vi "WILT Update State.vi"(10 "Station Number":i32, 11 "Station Test State In in":T1) -> (3 "Station Test State In out":T1)   [LabVIEW 2016]
uses:
  Type Definitions/WILT Station Test State Cluster.ctl
  Type Definitions/WILT Dryer Test State.ctl
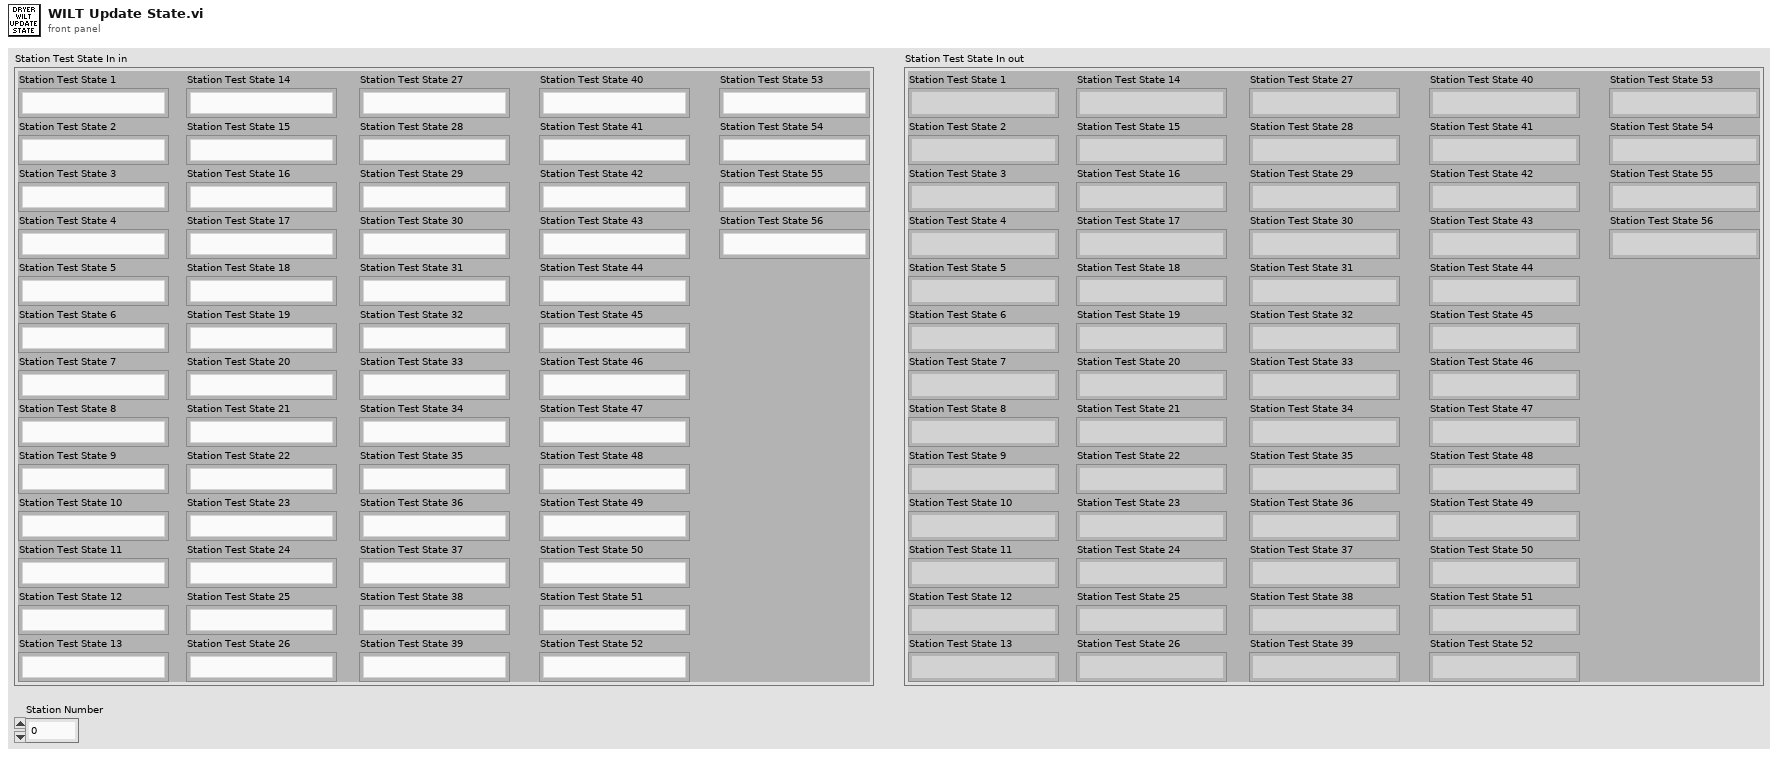
[diagram p1: front panel]
types:
  T1 = typedef "WILT Station Test State Cluster.ctl" = cluster{"Station Test State 1":T2, "Station Test State 2":T2, "Station Test State 3":T2, "Station Test State 4":T2, "Station Test State 5":T2, "Station Test State 6":T2, "Station Test State 7":T2, "Station Test State 8":T2, "Station Test State 9":T2, "Station Test State 10":T2, "Station Test State 11":T2, "Station Test State 12":T2, "Station Test State 13":T2, "Station Test State 14":T2, "Station Test State 15":T2, "Station Test State 16":T2, "Station Test State 17":T2, "Station Test State 18":T2, "Station Test State 19":T2, "Station Test State 20":T2, "Station Test State 21":T2, "Station Test State 22":T2, "Station Test State 23":T2, "Station Test State 24":T2, "Station Test State 25":T2, "Station Test State 26":T2, "Station Test State 27":T2, "Station Test State 28":T2, "Station Test State 29":T2, "Station Test State 30":T2, "Station Test State 31":T2, "Station Test State 32":T2, "Station Test State 33":T2, "Station Test State 34":T2, "Station Test State 35":T2, "Station Test State 36":T2, "Station Test State 37":T2, "Station Test State 38":T2, "Station Test State 39":T2, "Station Test State 40":T2, "Station Test State 41":T2, "Station Test State 42":T2, "Station Test State 43":T2, "Station Test State 44":T2, "Station Test State 45":T2, "Station Test State 46":T2, "Station Test State 47":T2, "Station Test State 48":T2, "Station Test State 49":T2, "Station Test State 50":T2, "Station Test State 51":T2, "Station Test State 52":T2, "Station Test State 53":T2, "Station Test State 54":T2, "Station Test State 55":T2, "Station Test State 56":T2}
  T2 = typedef "WILT Dryer Test State.ctl" = enum16{"No Serial Number", "Waiting for Dryer To Start", "Drying Clothes", "Water Injection 1 (On)", "Water Injection 1 Timer", "Water Injection 1 (Off)", "Pause Dryer", "Sending Start Stop CMD", "Pause Dryer 2", "Sending Start Stop CMD 2", "Drying Clothes 2", "Water Injection 2 (On)", "Water Injection 2 Timer", "Water Injection 2 (Off)", "Drying Clothes 3", "Cooling Down", "Sending Start Stop CMD 3", "Increment Cycle"}
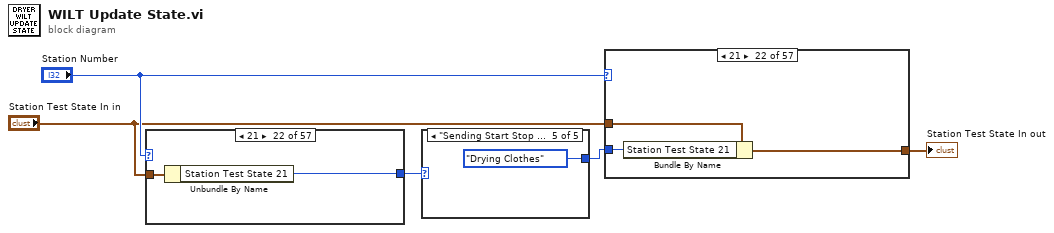
[diagram p0: block diagram]
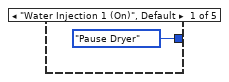
[diagram p2: hidden frame]
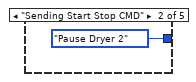
[diagram p3: hidden frame]
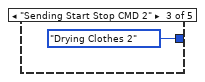
[diagram p4: hidden frame]
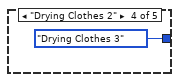
[diagram p5: hidden frame]
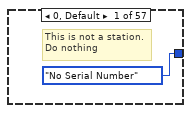
[diagram p6: hidden frame]
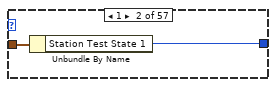
[diagram p7: hidden frame]
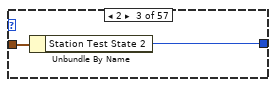
[diagram p8: hidden frame]
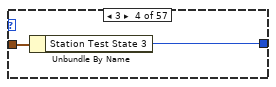
[diagram p9: hidden frame]
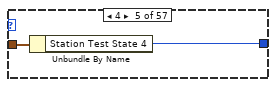
[diagram p10: hidden frame]
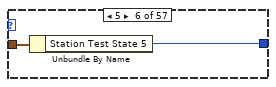
[diagram p11: hidden frame]
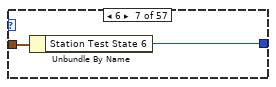
[diagram p12: hidden frame]
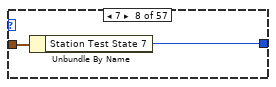
[diagram p13: hidden frame]
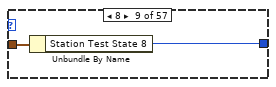
[diagram p14: hidden frame]
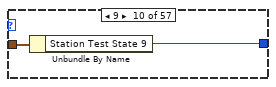
[diagram p15: hidden frame]
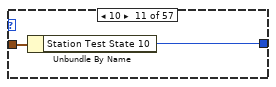
[diagram p16: hidden frame]
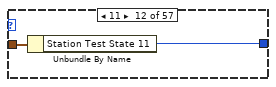
[diagram p17: hidden frame]
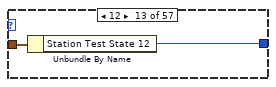
[diagram p18: hidden frame]
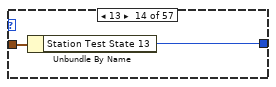
[diagram p19: hidden frame]
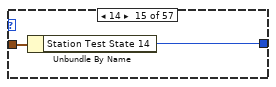
[diagram p20: hidden frame]
diagram:
  n1 = case shown="21" "Station Number" {
    tunnel: "Station Test State In in" -> [_ w8 w10 w12 w14 w16 w18 w20 w22 w24 w26 w28 w30 w32 w34 w36 w38 w40 w42 w44 w46 w48 w50 w52 w54 w56 w58 w60 w62 w64 w66 w68 w70 w72 w74 w76 w78 w80 w82 w84 w86 w88 w90 w92 w94 w96 w98 w100 w102 w104 w106 w108 w110 w112 w114 w116 w118]
    tunnel: [WILT_Dryer_Test_State."No Serial Number" ("Station Test State 56") w7 w9 w11 w13 w15 w17 w19 w21 w23 w25 w27 w29 w31 w33 w35 w37 w39 w41 w43 w45 w47 w49 w51 w53 w55 w57 w59 w61 w63 w65 w67 w69 w71 w73 w75 w77 w79 w81 w83 w85 w87 w89 w91 w93 w95 w97 w99 w101 w103 w105 w107 w109 w111 w113 w115 w117] -> w2
    frame 0, Default {
      # "This is not a station.\nDo nothing"
    }
    frame 1 {
      n2 = Unbundle By Name(w8) -> ("Station Test State 1"=w7:T2)
    }
    frame 2 {
      n3 = Unbundle By Name(w10) -> ("Station Test State 2"=w9:T2)
    }
    frame 3 {
      n4 = Unbundle By Name(w12) -> ("Station Test State 3"=w11:T2)
    }
    frame 4 {
      n5 = Unbundle By Name(w14) -> ("Station Test State 4"=w13:T2)
    }
    frame 5 {
      n6 = Unbundle By Name(w16) -> ("Station Test State 5"=w15:T2)
    }
    frame 6 {
      n7 = Unbundle By Name(w18) -> ("Station Test State 6"=w17:T2)
    }
    frame 7 {
      n8 = Unbundle By Name(w20) -> ("Station Test State 7"=w19:T2)
    }
    frame 8 {
      n9 = Unbundle By Name(w22) -> ("Station Test State 8"=w21:T2)
    }
    frame 9 {
      n10 = Unbundle By Name(w24) -> ("Station Test State 9"=w23:T2)
    }
    frame 10 {
      n11 = Unbundle By Name(w26) -> ("Station Test State 10"=w25:T2)
    }
    frame 11 {
      n12 = Unbundle By Name(w28) -> ("Station Test State 11"=w27:T2)
    }
    frame 12 {
      n13 = Unbundle By Name(w30) -> ("Station Test State 12"=w29:T2)
    }
    frame 13 {
      n14 = Unbundle By Name(w32) -> ("Station Test State 13"=w31:T2)
    }
    frame 14 {
      n15 = Unbundle By Name(w34) -> ("Station Test State 14"=w33:T2)
    }
    frame 15 {
      n16 = Unbundle By Name(w36) -> ("Station Test State 15"=w35:T2)
    }
    frame 16 {
      n17 = Unbundle By Name(w38) -> ("Station Test State 16"=w37:T2)
    }
    frame 17 {
      n18 = Unbundle By Name(w40) -> ("Station Test State 17"=w39:T2)
    }
    frame 18 {
      n19 = Unbundle By Name(w42) -> ("Station Test State 18"=w41:T2)
    }
    frame 19 {
      n20 = Unbundle By Name(w44) -> ("Station Test State 19"=w43:T2)
    }
    frame 20 {
      n21 = Unbundle By Name(w46) -> ("Station Test State 20"=w45:T2)
    }
    frame 21 {
      n22 = Unbundle By Name(w48) -> ("Station Test State 21"=w47:T2)
    }
    frame 22 {
      n23 = Unbundle By Name(w50) -> ("Station Test State 22"=w49:T2)
    }
    frame 23 {
      n24 = Unbundle By Name(w52) -> ("Station Test State 23"=w51:T2)
    }
    frame 24 {
      n25 = Unbundle By Name(w54) -> ("Station Test State 24"=w53:T2)
    }
    frame 25 {
      n26 = Unbundle By Name(w56) -> ("Station Test State 25"=w55:T2)
    }
    frame 26 {
      n27 = Unbundle By Name(w58) -> ("Station Test State 26"=w57:T2)
    }
    frame 27 {
      n28 = Unbundle By Name(w60) -> ("Station Test State 27"=w59:T2)
    }
    frame 28 {
      n29 = Unbundle By Name(w62) -> ("Station Test State 28"=w61:T2)
    }
    frame 29 {
      n30 = Unbundle By Name(w64) -> ("Station Test State 29"=w63:T2)
    }
    frame 30 {
      n31 = Unbundle By Name(w66) -> ("Station Test State 30"=w65:T2)
    }
    frame 31 {
      n32 = Unbundle By Name(w68) -> ("Station Test State 31"=w67:T2)
    }
    frame 32 {
      n33 = Unbundle By Name(w70) -> ("Station Test State 32"=w69:T2)
    }
    frame 33 {
      n34 = Unbundle By Name(w72) -> ("Station Test State 33"=w71:T2)
    }
    frame 34 {
      n35 = Unbundle By Name(w74) -> ("Station Test State 34"=w73:T2)
    }
    frame 35 {
      n36 = Unbundle By Name(w76) -> ("Station Test State 35"=w75:T2)
    }
    frame 36 {
      n37 = Unbundle By Name(w78) -> ("Station Test State 36"=w77:T2)
    }
    frame 37 {
      n38 = Unbundle By Name(w80) -> ("Station Test State 37"=w79:T2)
    }
    frame 38 {
      n39 = Unbundle By Name(w82) -> ("Station Test State 38"=w81:T2)
    }
    frame 39 {
      n40 = Unbundle By Name(w84) -> ("Station Test State 39"=w83:T2)
    }
    frame 40 {
      n41 = Unbundle By Name(w86) -> ("Station Test State 40"=w85:T2)
    }
    frame 41 {
      n42 = Unbundle By Name(w88) -> ("Station Test State 41"=w87:T2)
    }
    frame 42 {
      n43 = Unbundle By Name(w90) -> ("Station Test State 42"=w89:T2)
    }
    frame 43 {
      n44 = Unbundle By Name(w92) -> ("Station Test State 43"=w91:T2)
    }
    frame 44 {
      n45 = Unbundle By Name(w94) -> ("Station Test State 44"=w93:T2)
    }
    frame 45 {
      n46 = Unbundle By Name(w96) -> ("Station Test State 45"=w95:T2)
    }
    frame 46 {
      n47 = Unbundle By Name(w98) -> ("Station Test State 46"=w97:T2)
    }
    frame 47 {
      n48 = Unbundle By Name(w100) -> ("Station Test State 47"=w99:T2)
    }
    frame 48 {
      n49 = Unbundle By Name(w102) -> ("Station Test State 48"=w101:T2)
    }
    frame 49 {
      n50 = Unbundle By Name(w104) -> ("Station Test State 49"=w103:T2)
    }
    frame 50 {
      n51 = Unbundle By Name(w106) -> ("Station Test State 50"=w105:T2)
    }
    frame 51 {
      n52 = Unbundle By Name(w108) -> ("Station Test State 51"=w107:T2)
    }
    frame 52 {
      n53 = Unbundle By Name(w110) -> ("Station Test State 52"=w109:T2)
    }
    frame 53 {
      n54 = Unbundle By Name(w112) -> ("Station Test State 53"=w111:T2)
    }
    frame 54 {
      n55 = Unbundle By Name(w114) -> ("Station Test State 54"=w113:T2)
    }
    frame 55 {
      n56 = Unbundle By Name(w116) -> ("Station Test State 55"=w115:T2)
    }
    frame 56 {
      n57 = Unbundle By Name(w118) -> ("Station Test State 56"=w117:T2)
    }
  }
  n58 = case shown="\"Sending Start Stop CMD 3\"" w2 {
    tunnel: [WILT_Dryer_Test_State."Pause Dryer" ("Station Test State 56") WILT_Dryer_Test_State."Pause Dryer 2" ("Station Test State 56") WILT_Dryer_Test_State."Drying Clothes 2" ("Station Test State 56") WILT_Dryer_Test_State."Drying Clothes 3" ("Station Test State 56") WILT_Dryer_Test_State."Drying Clothes" ("Station Test State 56")] -> w3
    frame "Water Injection 1 (On)", Default {
    }
    frame "Sending Start Stop CMD" {
    }
    frame "Sending Start Stop CMD 2" {
    }
    frame "Drying Clothes 2" {
    }
    frame "Sending Start Stop CMD 3" {
    }
  }
  n59 = case shown="21" "Station Number" {
    tunnel: "Station Test State In in" -> [w124 w127 w130 w133 w136 w139 w142 w145 w148 w151 w154 w157 w160 w163 w166 w169 w172 w175 w178 w181 w184 w187 w190 w193 w196 w199 w202 w205 w208 w211 w214 w217 w220 w223 w226 w229 w232 w235 w238 w241 w244 w247 w250 w253 w256 w259 w262 w265 w268 w271 w274 w277 w280 w283 w286 w289 w292]
    tunnel: w3 -> [_ w126 w128 w131 w134 w137 w140 w143 w146 w149 w152 w155 w158 w161 w164 w167 w170 w173 w176 w179 w182 w185 w188 w191 w194 w197 w200 w203 w206 w209 w212 w215 w218 w221 w224 w227 w230 w233 w236 w239 w242 w245 w248 w251 w254 w257 w260 w263 w266 w269 w272 w275 w278 w281 w284 w287 w290]
    tunnel: [w124 w125 w129 w132 w135 w138 w141 w144 w147 w150 w153 w156 w159 w162 w165 w168 w171 w174 w177 w180 w183 w186 w189 w192 w195 w198 w201 w204 w207 w210 w213 w216 w219 w222 w225 w228 w231 w234 w237 w240 w243 w246 w249 w252 w255 w258 w261 w264 w267 w270 w273 w276 w279 w282 w285 w288 w291] -> w1
    frame 0, Default {
      # "Not a valid station. Do nothing"
    }
    frame 1 {
      n60 = Bundle By Name(cluster=w127, "Station Test State 1"=w126) -> (w125:T1)
    }
    frame 2 {
      n61 = Bundle By Name(cluster=w130, "Station Test State 2"=w128) -> (w129:T1)
    }
    frame 3 {
      n62 = Bundle By Name(cluster=w133, "Station Test State 3"=w131) -> (w132:T1)
    }
    frame 4 {
      n63 = Bundle By Name(cluster=w136, "Station Test State 4"=w134) -> (w135:T1)
    }
    frame 5 {
      n64 = Bundle By Name(cluster=w139, "Station Test State 5"=w137) -> (w138:T1)
    }
    frame 6 {
      n65 = Bundle By Name(cluster=w142, "Station Test State 6"=w140) -> (w141:T1)
    }
    frame 7 {
      n66 = Bundle By Name(cluster=w145, "Station Test State 7"=w143) -> (w144:T1)
    }
    frame 8 {
      n67 = Bundle By Name(cluster=w148, "Station Test State 8"=w146) -> (w147:T1)
    }
    frame 9 {
      n68 = Bundle By Name(cluster=w151, "Station Test State 9"=w149) -> (w150:T1)
    }
    frame 10 {
      n69 = Bundle By Name(cluster=w154, "Station Test State 10"=w152) -> (w153:T1)
    }
    frame 11 {
      n70 = Bundle By Name(cluster=w157, "Station Test State 11"=w155) -> (w156:T1)
    }
    frame 12 {
      n71 = Bundle By Name(cluster=w160, "Station Test State 12"=w158) -> (w159:T1)
    }
    frame 13 {
      n72 = Bundle By Name(cluster=w163, "Station Test State 13"=w161) -> (w162:T1)
    }
    frame 14 {
      n73 = Bundle By Name(cluster=w166, "Station Test State 14"=w164) -> (w165:T1)
    }
    frame 15 {
      n74 = Bundle By Name(cluster=w169, "Station Test State 15"=w167) -> (w168:T1)
    }
    frame 16 {
      n75 = Bundle By Name(cluster=w172, "Station Test State 16"=w170) -> (w171:T1)
    }
    frame 17 {
      n76 = Bundle By Name(cluster=w175, "Station Test State 17"=w173) -> (w174:T1)
    }
    frame 18 {
      n77 = Bundle By Name(cluster=w178, "Station Test State 18"=w176) -> (w177:T1)
    }
    frame 19 {
      n78 = Bundle By Name(cluster=w181, "Station Test State 19"=w179) -> (w180:T1)
    }
    frame 20 {
      n79 = Bundle By Name(cluster=w184, "Station Test State 20"=w182) -> (w183:T1)
    }
    frame 21 {
      n80 = Bundle By Name(cluster=w187, "Station Test State 21"=w185) -> (w186:T1)
    }
    frame 22 {
      n81 = Bundle By Name(cluster=w190, "Station Test State 22"=w188) -> (w189:T1)
    }
    frame 23 {
      n82 = Bundle By Name(cluster=w193, "Station Test State 23"=w191) -> (w192:T1)
    }
    frame 24 {
      n83 = Bundle By Name(cluster=w196, "Station Test State 24"=w194) -> (w195:T1)
    }
    frame 25 {
      n84 = Bundle By Name(cluster=w199, "Station Test State 25"=w197) -> (w198:T1)
    }
    frame 26 {
      n85 = Bundle By Name(cluster=w202, "Station Test State 26"=w200) -> (w201:T1)
    }
    frame 27 {
      n86 = Bundle By Name(cluster=w205, "Station Test State 27"=w203) -> (w204:T1)
    }
    frame 28 {
      n87 = Bundle By Name(cluster=w208, "Station Test State 28"=w206) -> (w207:T1)
    }
    frame 29 {
      n88 = Bundle By Name(cluster=w211, "Station Test State 29"=w209) -> (w210:T1)
    }
    frame 30 {
      n89 = Bundle By Name(cluster=w214, "Station Test State 30"=w212) -> (w213:T1)
    }
    frame 31 {
      n90 = Bundle By Name(cluster=w217, "Station Test State 31"=w215) -> (w216:T1)
    }
    frame 32 {
      n91 = Bundle By Name(cluster=w220, "Station Test State 32"=w218) -> (w219:T1)
    }
    frame 33 {
      n92 = Bundle By Name(cluster=w223, "Station Test State 33"=w221) -> (w222:T1)
    }
    frame 34 {
      n93 = Bundle By Name(cluster=w226, "Station Test State 34"=w224) -> (w225:T1)
    }
    frame 35 {
      n94 = Bundle By Name(cluster=w229, "Station Test State 35"=w227) -> (w228:T1)
    }
    frame 36 {
      n95 = Bundle By Name(cluster=w232, "Station Test State 36"=w230) -> (w231:T1)
    }
    frame 37 {
      n96 = Bundle By Name(cluster=w235, "Station Test State 37"=w233) -> (w234:T1)
    }
    frame 38 {
      n97 = Bundle By Name(cluster=w238, "Station Test State 38"=w236) -> (w237:T1)
    }
    frame 39 {
      n98 = Bundle By Name(cluster=w241, "Station Test State 39"=w239) -> (w240:T1)
    }
    frame 40 {
      n99 = Bundle By Name(cluster=w244, "Station Test State 40"=w242) -> (w243:T1)
    }
    frame 41 {
      n100 = Bundle By Name(cluster=w247, "Station Test State 41"=w245) -> (w246:T1)
    }
    frame 42 {
      n101 = Bundle By Name(cluster=w250, "Station Test State 42"=w248) -> (w249:T1)
    }
    frame 43 {
      n102 = Bundle By Name(cluster=w253, "Station Test State 43"=w251) -> (w252:T1)
    }
    frame 44 {
      n103 = Bundle By Name(cluster=w256, "Station Test State 44"=w254) -> (w255:T1)
    }
    frame 45 {
      n104 = Bundle By Name(cluster=w259, "Station Test State 45"=w257) -> (w258:T1)
    }
    frame 46 {
      n105 = Bundle By Name(cluster=w262, "Station Test State 46"=w260) -> (w261:T1)
    }
    frame 47 {
      n106 = Bundle By Name(cluster=w265, "Station Test State 47"=w263) -> (w264:T1)
    }
    frame 48 {
      n107 = Bundle By Name(cluster=w268, "Station Test State 48"=w266) -> (w267:T1)
    }
    frame 49 {
      n108 = Bundle By Name(cluster=w271, "Station Test State 49"=w269) -> (w270:T1)
    }
    frame 50 {
      n109 = Bundle By Name(cluster=w274, "Station Test State 50"=w272) -> (w273:T1)
    }
    frame 51 {
      n110 = Bundle By Name(cluster=w277, "Station Test State 51"=w275) -> (w276:T1)
    }
    frame 52 {
      n111 = Bundle By Name(cluster=w280, "Station Test State 52"=w278) -> (w279:T1)
    }
    frame 53 {
      n112 = Bundle By Name(cluster=w283, "Station Test State 53"=w281) -> (w282:T1)
    }
    frame 54 {
      n113 = Bundle By Name(cluster=w286, "Station Test State 54"=w284) -> (w285:T1)
    }
    frame 55 {
      n114 = Bundle By Name(cluster=w289, "Station Test State 55"=w287) -> (w288:T1)
    }
    frame 56 {
      n115 = Bundle By Name(cluster=w292, "Station Test State 56"=w290) -> (w291:T1)
    }
  }
  "Station Test State In out" <- w1
